vi "Z900_navX_Set_ZeroYaw.vi"(8 "error in (no error)":errorcluster, 11 "navX Device":T1={"Interface"={"Protocol"=enum."SERIAL", "Update Rate (4Hz-100Hz)"=4, "navX Open TypeDef"=variant}, "Notify Packet"=refnum, "Loop VI Refnum"=refnum, "Ready to Close Occurrence Refnum"=refnum} {"Interface"."Update Rate (4Hz-100Hz)" min=4 max=60 step=1}) -> (0 "error out":errorcluster, 3 "navX Device":T1={"Interface"={"Protocol"=enum."SERIAL", "Update Rate (4Hz-100Hz)"=4, "navX Open TypeDef"=variant}, "Notify Packet"=refnum, "Loop VI Refnum"=refnum, "Ready to Close Occurrence Refnum"=refnum} {"Interface"."Update Rate (4Hz-100Hz)" min=4 max=60 step=1})   [LabVIEW 2016, in "navX Library v2.lvlib"]
doc: "This navX VI will zero the navX yaw."
uses:
  navX Library v2.lvlib
  TypeDefs/Z900_navX_DeviceTypeDef.ctl
  TypeDefs/Z900_navX_ProtocolTypeDef.ctl
  TypeDefs/Z900_navX_NotifyPacketTypeDef.ctl
  TypeDefs/Z900_navX_ActionTypeDef.ctl
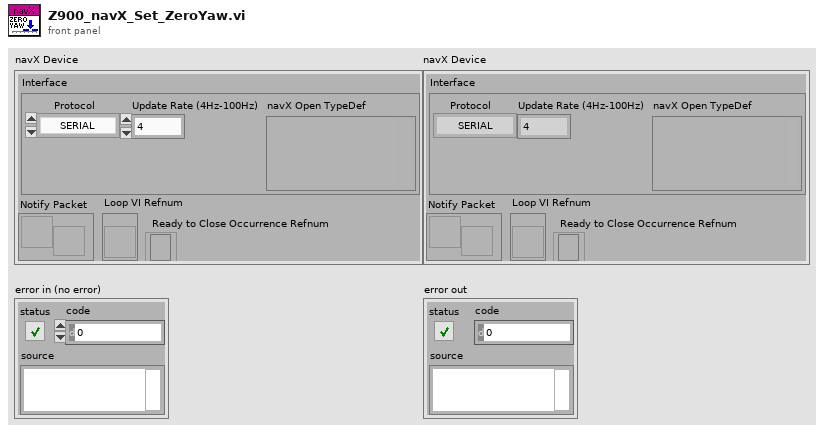
[diagram p1: front panel]
types:
  T1 = typedef "navX Library v2.lvlib/Z900_navX_DeviceTypeDef.ctl" = cluster{"Interface":cluster{"Protocol":T2, "Update Rate (4Hz-100Hz)":u8, "navX Open TypeDef":variant}, "Notify Packet":refnum<notifier>, "Loop VI Refnum":refnum<vi>, "Ready to Close Occurrence Refnum":refnum<k4>}
  T2 = typedef "navX Library v2.lvlib/Z900_navX_ProtocolTypeDef.ctl" = enum16{"SERIAL", "I2C", "SPI"}
  T3 = typedef "navX Library v2.lvlib/Z900_navX_ActionTypeDef.ctl" = enum16{"None", "Halt", "Update Serial Protocol", "Zero-Yaw", "Zero-Displacement", "Zero-Velocity"}
  T4 = typedef "navX Library v2.lvlib/Z900_navX_NotifyPacketTypeDef.ctl" = cluster{"navX Action":T3, "Data":variant}
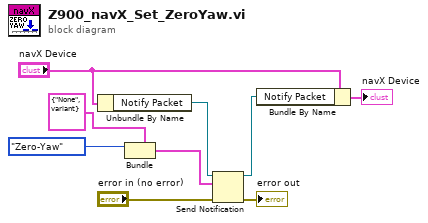
[diagram p0: block diagram]
diagram:
  n1 = Unbundle By Name("navX Device") -> ("Notify Packet"=w9:refnum<notifier>)
  n2 = Bundle(cluster=T4 {"navX Action"=enum."None", "Data"=variant} ("navX Notify Packet"), "navX Action"=Z900_navX_ActionTypeDef."Zero-Yaw") -> (w2:T4)  [unwired: 1 in]
  n3 = Send Notification(notification=w2, notifier=w9, error in (no error)="error in (no error)") -> (notifier out=w7:refnum<notifier>, error out=→"error out":errorcluster)
  n4 = Bundle By Name(cluster="navX Device", "Notify Packet"=w7) -> (→"navX Device":T1)
